vi "sub_Gslam.vi"(10 "hz":dbl[][][](array[numeric]), 11 "hxDR":cluster{"x":dbl, "y":dbl, "yaw":dbl}[](array[cluster])) -> (3 "x_opt out":cluster{"x":dbl, "y":dbl, "yaw":dbl}[](array[cluster]))   [LabVIEW 2019]
uses:
  Ctrl/cmd_common.ctl
  Ctrl/cmd_ini-RW.ctl
  <vilib>/Analysis/Matrix/Numeric/Conversions/Array To Matrix - RA2.vi
  <vilib>/Analysis/Matrix/Numeric/Conversions/Array To Matrix - RA.vi
  <vilib>/Analysis/Matrix/Numeric/Add/Add - RM,RM.vi
  <vilib>/Analysis/baseanly.llb/Real Inverse Matrix.vi
  <vilib>/Analysis/Matrix/Numeric/Multiply/Multiply - RM,RM.vi
  <vilib>/Analysis/Matrix/Numeric/Conversions/Matrix To Array - RM.vi
  <vilib>/Analysis/Matrix/NI_Matrix.lvlib
  <vilib>/Analysis/NI_AALBase.lvlib
panel:
  out "x_opt graph":cluster{"X":dbl, "Y":dbl}[](graph)
  out "H update1":dbl[][](graph)
  out "i2":i32
  out "i1":i32
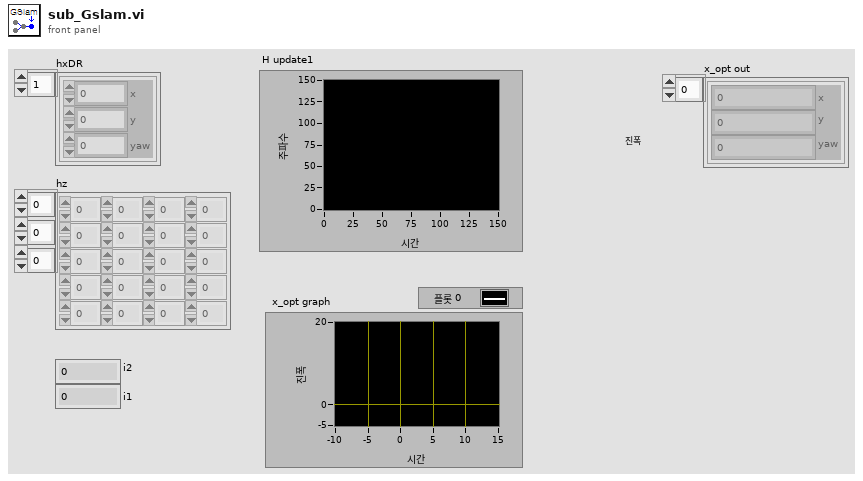
[diagram p1: front panel]
types:
  T1 = typedef "cmd_common.ctl" = enum16{"read", "write"}
  T2 = typedef "cmd_ini-RW.ctl" = enum16{"ini", "read", "write"}
  T3 = typedef "NI_Matrix.lvlib/RealMatrix.ctl" = dbl[][]
  T4 = cluster{"Q Sim":T3, "R Sim":T3, "DT":dbl, "SIM_TIME":dbl, "MAX_RANGE":dbl, "STATE_SIZE":i32, "C_SIGMA 1":dbl, "C_SIGMA 2":dbl, "C_SIGMA 3":dbl, "MAX_ITR":u32}
  T5 = cluster{"e":T3, "omega":T3, "d1":dbl, "d2":dbl, "yaw1":dbl, "yaw2":dbl, "angle1":dbl, "angle2":dbl, "id1":i32, "id2":i32}[]
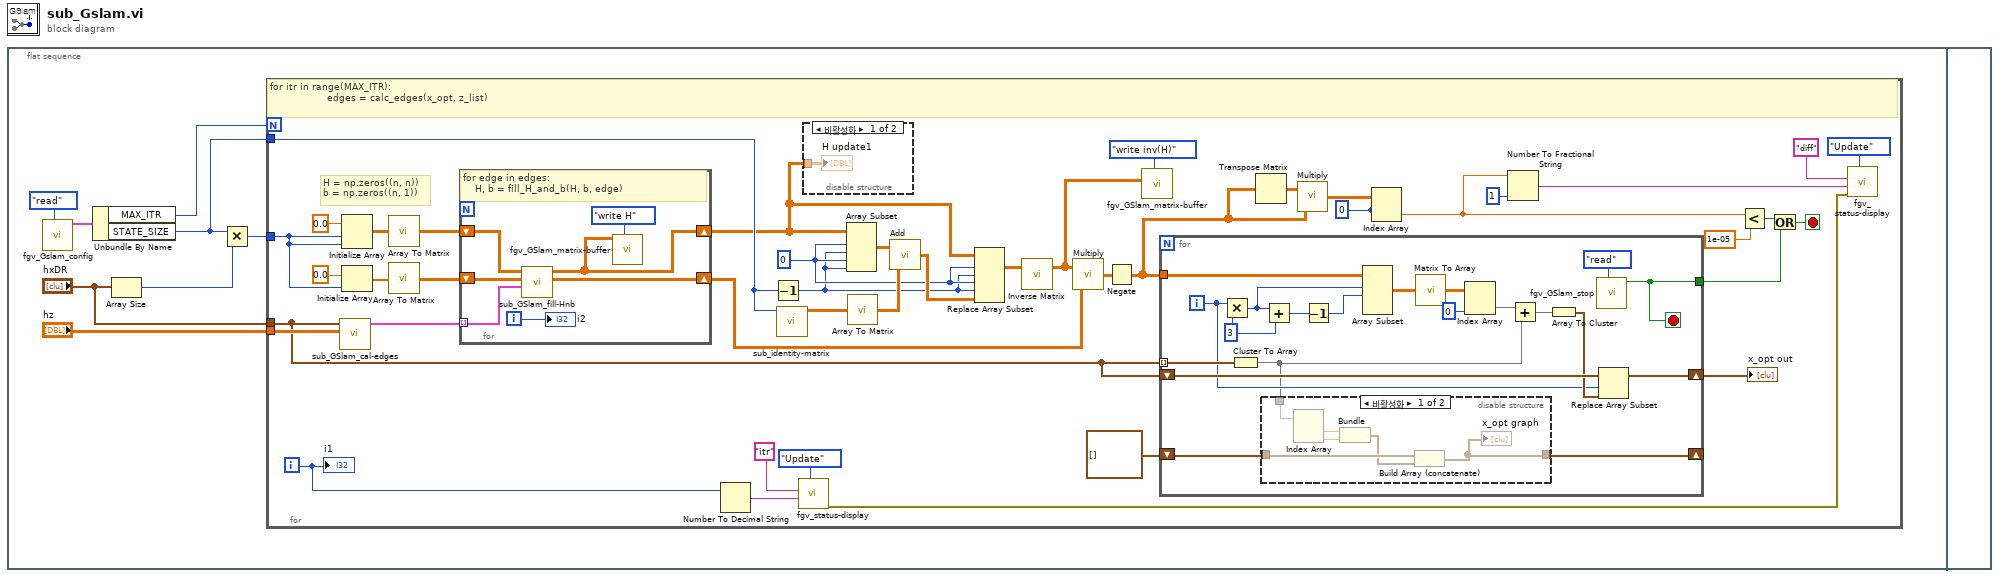
[diagram p0: block diagram]
diagram:
  n1 = flat-sequence {
    frame #0 {
      n2 = call "fgv_Gslam_config.vi"("cmd"=cmd_common."read") -> ("G cofnig out"=w7:T4)  [unwired: 10 in]
      n3 = Unbundle By Name(w7) -> ("MAX_ITR"=w5:u32, "STATE_SIZE"=w2:i32)
      n4 = Array Size(array="hxDR") -> (size(s)=w1:i32)
      n5 = Multiply(x=w2, y=w1) -> (x*y=w4:i32)
      n6 = for {
        N: w5 -> [_]
        tunnel: "hz" -> [w51]
        tunnel: "hxDR" -> [w35]
        tunnel: w4 -> [w48]
        tunnel: w2 -> [w33]
        i -> [w15]
        stop <- w10 stop-if-true
        w28 = 0 ("인덱스 (행)")
        w38 = 0 ("행 1")
        # "H = np.zeros((n, n))\nb = np.zeros((n, 1))"
        # "for itr in range(MAX_ITR):\n                   edges = calc_edges(x_opt, z_list)"
        n7 = call "sub_GSlam_cal-edges.vi"("z_list"=w51, "x_list"=w35) -> ("edge arr"=w45:T5)  [unwired: 8 in, 1 out]
        n8 = Initialize Array(0.0 ("원소"), w48, w48) -> (w47:dbl[][])
        n9 = Initialize Array(0.0 ("원소"), w48) -> (w46:dbl[])
        n10 = call-poly <vilib>:"Array To Matrix.vi"("Real 2D Array"=w47) -> ("Real Matrix"=w44:T3)
        n11 = call-poly <vilib>:"Array To Matrix.vi"("Real 1D Array"=w46) -> ("Real Matrix (Column Vector)"=w43:T3)
        n12 = for {
          tunnel: w45 -> [w84] mode=indexing
          shift-right: [w79] -> w22
          shift-left: w44 -> [w81]
          shift-right: [w83] -> w36
          shift-left: w43 -> [w85]
          i -> [w82]
          # "for edge in edges:\n    H, b = fill_H_and_b(H, b, edge)"
          n13 = call "sub_GSlam_fill-Hnb.vi"("edge in"=w84, "b"=w85, "H"=w81) -> ("b out"=w83:T3, "H out"=w79:T3)  [unwired: 7 in]
          n14 = call "fgv_GSlam_matrix-buffer.vi"("cmd"=enum16{"write H", "write inv(H)", "read"}."write H", "H"=w79) -> ()  [unwired: 8 in, 2 out]
          "i2" <- w82
        }
        n15 = Number To Decimal String(number=w15) -> (decimal integer string=w14:string)  [unwired: 1 in]
        n16 = Decrement(x=w33) -> (x-1=w34:i32)
        n17 = call "sub_identity-matrix.vi"("STATE_SIZE"=w33) -> ("identity"=w41:dbl[][])  [unwired: 10 in]
        n18 = call "fgv_status-display.vi"("Mode"=enum16{"Initial", "Update", "Clear"}."Update", "detail"=w14, "title"="itr") -> ("error out"=w13:errorcluster)  [unwired: 8 in]
        n19 = disable-structure shown="비활성화" {
          disable-tunnel: w22 -> [w52 _]
          frame Disabled {
            "H update1" <- w52
          }
          frame Enabled {
          }
        }
        n20 = Array Subset(array=w22, index (row)=w38, length (row)=w34, index (col)=w38, length (col)=w34) -> (w42:T3)
        n21 = call-poly <vilib>:"Array To Matrix.vi"("Real 2D Array"=w41) -> ("Real Matrix"=w40:T3)
        n22 = call-poly <vilib>:"Add.vi"("Real Matrix B"=w40, "Real Matrix A"=w42) -> ("A + B"=w39:T3)
        n23 = Replace Array Subset(array=w22, new element=w39, index (dim 0)=w38, index (dim 1)=w34, index (dim 2)=w38, index (dim 3)=w34) -> (w32:T3)
        n24 = call-poly <vilib>:"Inverse Matrix.vi"("Input Matrix"=w32) -> ("Inverse Matrix"=w23:T3)  [unwired: 1 in, 1 out]
        n25 = call-poly <vilib>:"Multiply.vi"("Real Matrix B"=w36, "Real Matrix A"=w23) -> ("A * B"=w37:T3)
        n26 = Negate(x=w37) -> (-x=w30:T3)
        n27 = call "fgv_GSlam_matrix-buffer.vi"("cmd"=enum16{"write H", "write inv(H)", "read"}."write inv(H)", "H inv"=w23) -> ()  [unwired: 8 in, 2 out]
        n28 = for {
          shift-right: [w59] -> w26
          shift-left: w35 -> [w62]
          tunnel: w35 -> [w68] mode=indexing
          tunnel: w30 -> [w71]
          shift-right: [w55] -> _
          shift-left: cluster{"x":dbl, "x":dbl}[] [] -> [w56]
          tunnel: [w53] -> w9
          i -> [w58]
          stop <- w53 stop-if-true
          w72 = 3 ("y")
          n29 = Multiply(x=w58, y=w72) -> (x*y=w61:i32)
          n30 = Cluster To Array(cluster=w68) -> (array=w57:dbl[])
          n31 = disable-structure shown="비활성화" {
            disable-tunnel: w57 -> [w78 _]
            disable-tunnel: w56 -> [w75 _]
            disable-tunnel: [w73 _] -> w55
            frame Disabled {
              n32 = Index Array(array=w78) -> (element #1=w76:dbl, element #2=w77:dbl)  [unwired: 2 in]
              n33 = Bundle("x"=w76, "x"=w77) -> (w74:cluster{"x":dbl, "x":dbl})  [unwired: 1 in]
              n34 = Build Array (concatenate)(w75, w74) -> (w73:cluster{"x":dbl, "x":dbl}[])
              "x_opt graph" <- w73
            }
            frame Enabled {
            }
          }
          n35 = Add(x=w61, y=w72) -> (x+y=w70:i32)
          n36 = Decrement(x=w70) -> (x-1=w69:i32)
          n37 = Array Subset(array=w71, index (row)=w61, length (row)=w69) -> (w67:T3)  [unwired: 2 in]
          n38 = call-poly <vilib>:"Matrix To Array.vi"("Real Matrix"=w67) -> ("Real 2D Array"=w66:dbl[][])
          n39 = Index Array(array=w66, index (col)=0 ("비활성화된 인덱스 (열)")) -> (element=w64:dbl[])  [unwired: 1 in]
          n40 = Add ("Add.vi")(x=w64, y=w57) -> (x+y=w63:dbl[])
          n41 = Array To Cluster(array=w63) -> (cluster=w60:cluster{"[0]":dbl, "[1]":dbl, "[2]":dbl})
          n42 = call "fgv_GSlam_stop.vi"("cmd"=cmd_ini-RW."read") -> ("val"=w53:bool)  [unwired: 10 in]
          n43 = Replace Array Subset(array=w62, new element=w60, index=w58) -> (w59:cluster{"x":dbl, "y":dbl, "yaw":dbl}[])
        }
        "x_opt out" <- w26
        n44 = Transpose Matrix(1:w30) -> (0:w31:T3)
        n45 = call-poly <vilib>:"Multiply.vi"("Real Matrix B"=w30, "Real Matrix A"=w31) -> ("A * B"=w29:T3)
        n46 = Index Array(array=w29, index (row)=w28, index (col)=w28) -> (element=w20:dbl)
        n47 = Number To Fractional String(number=w20, precision (6)=i16 1 ("정밀도(6)")) -> (F-format string=w19:string)  [unwired: 2 in]
        n48 = Less?(x=w20, y=1e-05) -> (x < y?=w11:bool)
        n49 = Or(x=w11, y=w9) -> (x .or. y?=w10:bool)
        n50 = call "fgv_status-display.vi"("Mode"=enum16{"Initial", "Update", "Clear"}."Update", "error in"=w13, "detail"=w19, "title"="diff") -> ()  [unwired: 7 in, 1 out]
        "i1" <- w15
      }
    }
    frame #1 {
    }
  }
